vi "Initialize.vi"(8 "error in (no error)":errorcluster, 10 "Settings":variant, 11 "Base Hardware in":refnum<class "Base Hardware.lvclass">) -> (0 "error out":errorcluster, 3 "Base Hardware out":refnum<class "Base Hardware.lvclass">)   [LabVIEW 2023, in "Abstract Hardware.lvlib" / "Base Hardware.lvclass"]
uses:
  Base Hardware.lvclass
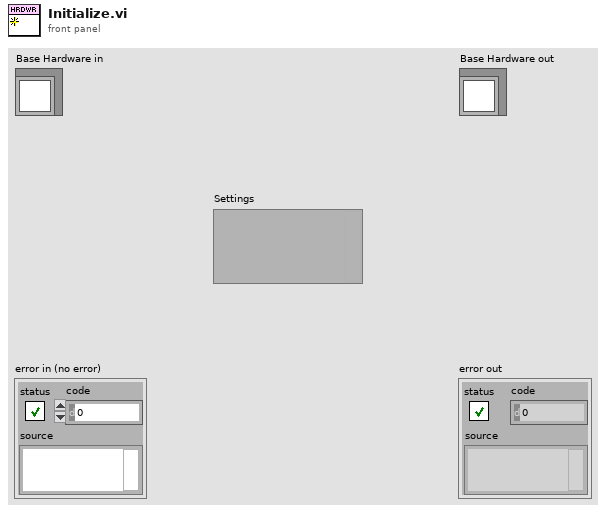
[diagram p1: front panel]
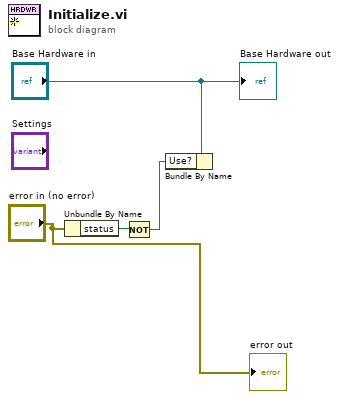
[diagram p0: block diagram]
diagram:
  n1 = Unbundle By Name("error in (no error)") -> ("status"=w3:bool)
  n2 = Not(x=w3) -> (.not. x?=w2:bool)
  n3 = Bundle By Name(cluster="Base Hardware in", "Use?"=w2) -> ()  [unwired: 1 out]
  "error out" <- "error in (no error)"
  "Base Hardware out" <- "Base Hardware in"
